vi "Configure Modulation (Phase).vi"(0 "VISA resource name":refnum<visa-resource-name>, 1 "Enable Phase Modulation (T: Enable)":bool=TRUE, 2 "File Path":string, 5 "Channel (0: Channel 1)":u16(ring) items=["Channel 1", "Channel 2"], 7 "PM Source (0: Internal)":u16(ring) items=["Internal", "External"], 9 "Modulation Waveform (0: Sine)":u16(ring) items=["Sine", "Square", "Triangle", "Ramp", "Down Ramp", "Noise", "User 1", "User 2", "User 3", "User 4", "Edit Memory", "Edit Path"], 11 "error in (no error)":errorcluster, 12 "Modulation Frequency (100.00 Hz)":dbl=100.0 format="%#_6f", 13 "Peak Deviation (90 deg)":dbl=90.0 min=-180.0 max=180.0 format="%#.4f") -> (4 "VISA resource name out":refnum<visa-resource-name>, 15 "error out":errorcluster)   [LabVIEW 2015, in "Tektronix AFG 3000 Series.lvlib"]
doc: "Configures and enables phase modulation (PM). In PM, the phase of the carrier is varied by the peak deviation and the modulating waveform.\n\n<B>Note:</B>\n\nDefault measure for peak deviation is in degrees only. To change deviation unit to radians replace the DEG with RAD in the peak deviation command."
uses:
  Tektronix AFG 3000 Series.lvlib
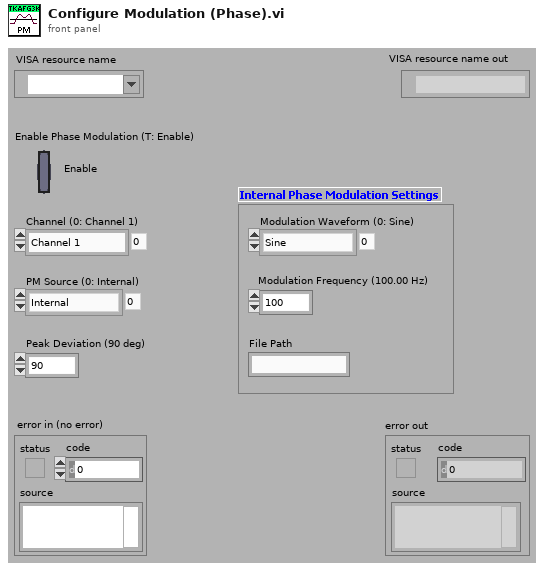
[diagram p1: front panel]
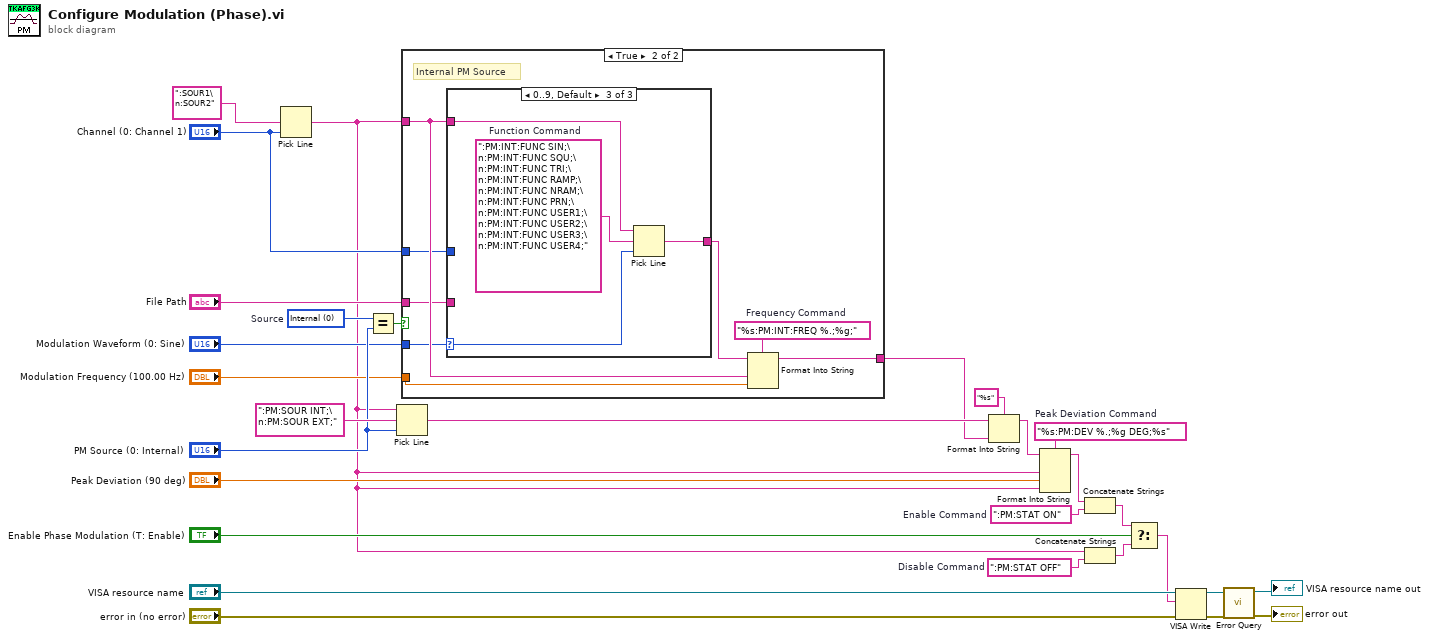
[diagram p0: block diagram]
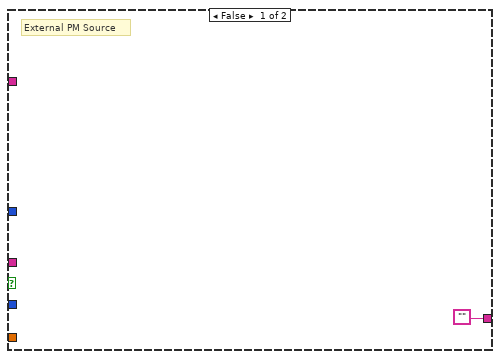
[diagram p2: hidden frame]
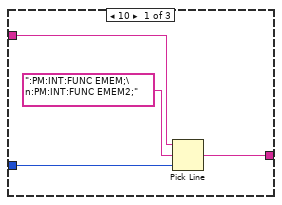
[diagram p3: hidden frame]
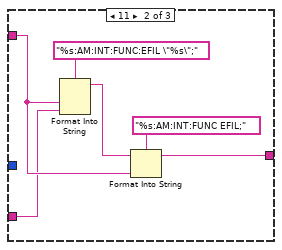
[diagram p4: hidden frame]
diagram:
  w21 = ":PM:STAT ON"  # Enable Command
  w23 = "%s:PM:DEV %.;%g DEG;%s"  # Peak Deviation Command
  w4 = u16 0 items=["Internal", "External"]  # Source
  w18 = ":PM:STAT OFF"  # Disable Command
  n1 = Pick Line(multi-line string=":SOUR1\n:SOUR2" ("string (\"\")"), line index="Channel (0: Channel 1)") -> (output string=w1:string)  [unwired: 1 in]
  n2 = Equal?(x=w4, y="PM Source (0: Internal)") -> (x = y?=w12:bool)
  n3 = Pick Line(string ("")=w1, multi-line string=":PM:SOUR INT;\n:PM:SOUR EXT;" ("Source Command"), line index="PM Source (0: Internal)") -> (output string=w9:string)
  n4 = case shown="True" w12 {
    tunnel: ["" w37] -> w8
    tunnel: w1 -> [_ w35]
    tunnel: "Modulation Waveform (0: Sine)" -> [_ w33]
    tunnel: "Modulation Frequency (100.00 Hz)" -> [_ w36]
    tunnel: "File Path" -> [_ w34]
    tunnel: "Channel (0: Channel 1)" -> [_ w32]
    frame False {
      # "External PM Source"
    }
    frame True {
      w38 = "%s:PM:INT:FREQ %.;%g;"  # Frequency Command
      # "Internal PM Source"
      n5 = case shown="0..9, Default" w33 {
        selector: w33 -> [_ _ w50]
        tunnel: w35 -> [w41 w46 w51]
        tunnel: w32 -> [w40 _ _]
        tunnel: w34 -> [_ w45 _]
        tunnel: [w39 w43 w49] -> w31
        frame 10 {
          n6 = Pick Line(string ("")=w41, multi-line string=":PM:INT:FUNC EMEM;\n:PM:INT:FUNC EMEM2;", line index=w40) -> (output string=w39:string)
        }
        frame 11 {
          n7 = Format Into String(format string="%s:AM:INT:FUNC:EFIL \"%s\";", w46, w45) -> (resulting string=w48:string)  [unwired: 2 in, 1 out]
          n8 = Format Into String(format string="%s:AM:INT:FUNC EFIL;", initial string=w48, w46) -> (resulting string=w43:string)  [unwired: 1 in, 1 out]
        }
        frame 0..9, Default {
          w52 = ":PM:INT:FUNC SIN;\n:PM:INT:FUNC SQU;\n:PM:INT:FUNC TRI;\n:PM:INT:FUNC RAMP;\n:PM:INT:FUNC NRAM;\n:PM:INT:FUNC PRN;\n:PM:INT:FUNC USER1;\n:PM:INT:FUNC USER2;\n:PM:INT:FUNC USER3;\n:PM:INT:FUNC USER4;"  # Function Command
          n9 = Pick Line(string ("")=w51, multi-line string=w52, line index=w50) -> (output string=w49:string)
        }
      }
      n10 = Format Into String(format string=w38, initial string=w31, w35, w36) -> (resulting string=w37:string)  [unwired: 1 in, 1 out]
    }
  }
  n11 = Format Into String(format string="%s", initial string=w9, w8) -> (resulting string=w7:string)  [unwired: 1 in, 1 out]
  n12 = Format Into String(format string=w23, initial string=w7, w1, "Peak Deviation (90 deg)", w1) -> (resulting string=w22:string)  [unwired: 1 in, 1 out]
  n13 = Concatenate Strings(w22, w21) -> (w15:string)
  n14 = Concatenate Strings(w1, w18) -> (w16:string)
  n15 = Select(t=w15, s="Enable Phase Modulation (T: Enable)", f=w16) -> (s? t:f=w14:string)
  n16 = VISA Write(VISA resource name="VISA resource name", write buffer=w14, error in (no error)="error in (no error)") -> (VISA resource name out=w27:refnum<visa-resource-name>, error out=w26:errorcluster)  [unwired: 1 out]
  n17 = call "Error Query.vi"("error in (no error)"=w26, "VISA resource name"=w27) -> ("error out"=→"error out":errorcluster, "VISA resource name out"=→"VISA resource name out":refnum<visa-resource-name>)  [unwired: 6 in, 2 out]
